vi "06_2.vi"() -> ()   [LabVIEW 2018]
uses:
  <userlib>/_OpenG.lib/array/array.llb/Search 1D Array (U8)__ogtk.vi
panel:
  out "sum":i16
  in  "String":string="wzaopvscxknyjtiul\nbelforsgdhuvmwc\n\nkiocpzjhsetqnwbl\nmaciywlbpodgevujnsktrz\nkpebjfchtlsonwiz\npcezwjtsinxlobk\n\nlrcp\ncdlbepr\nrlqcyutp\nlcpr\nlrtcpym\n\ngxcqbowaelfjhpknz\ngflhackzwqxojeb\nlfwocexqbkjhgaz\n\nfpivaozqnkextmbrjhycdwug\nmotgcrzaisqlpdwbeyhukf\nhbiqcdmkpawueyztgfor\nzrcehkqyoblmtgfiaupdw\n\numjz\njzu\nvzowkpuj\njmzau\n\nunzlx\nlnzxu\nmxluzn\nnzuxli\n\nszkiauhyntdrbcljomqwepv\namowcpzbyukihsjtqelnd\nlzctuqjabmsynphkewxido\nsikblhptcoqemdanywzju\njdeiylutspabcwngfzqkhom\n\nzgyhwtnxjdqucbp\nptnzhudjbcxgkqf\nzgqhjbdnutcmpx\ngjbzhpdxanqcut\n\nwjkcsqlu\nucsjq\n\nvkzsqtunmr\nljcexadhg\n\nfhtrusba\nsvtk\npgzwytn\nastb\n\nhvzjiwlsmnatbxg..."
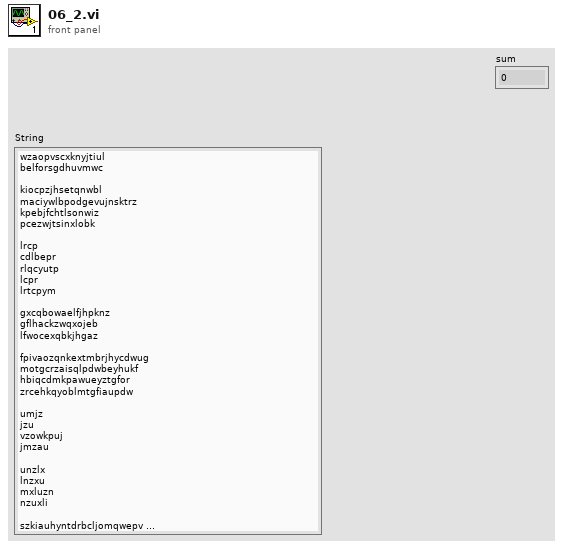
[diagram p1: front panel]
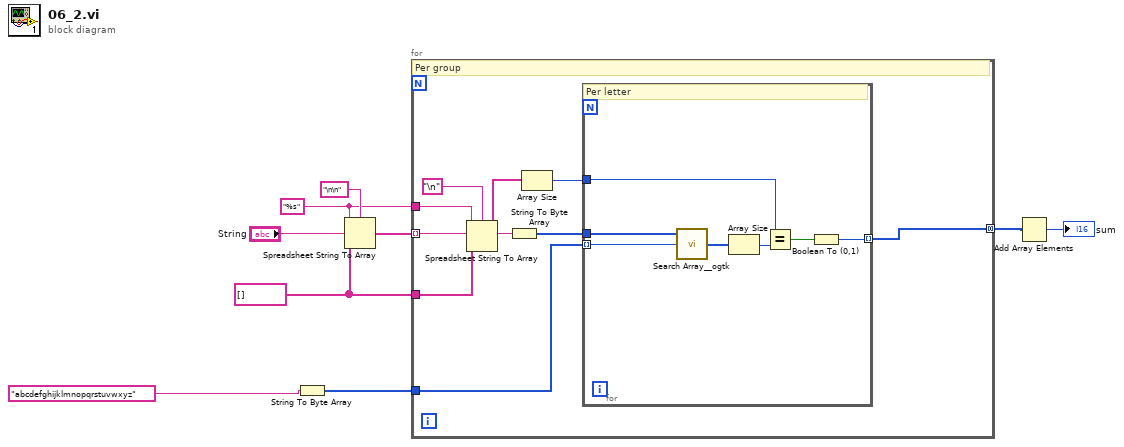
[diagram p0: block diagram]
diagram:
  w3 = string[] []
  w4 = "%s"
  n1 = String To Byte Array(string="abcdefghijklmnopqrstuvwxyz") -> (unsigned byte array=w1:u8[])
  n2 = Spreadsheet String To Array(delimiter (Tab)="\n\n", format string=w4, spreadsheet string="String", array type (2D Dbl)=w3) -> (array=w7:string[])
  n3 = for {
    tunnel: w7 -> [w14] mode=indexing
    tunnel: [w11] -> w6 mode=concatenating
    tunnel: w4 -> [w18]
    tunnel: w3 -> [w16]
    tunnel: w1 -> [w10]
    # "Per group"
    n4 = Spreadsheet String To Array(delimiter (Tab)="\n", format string=w18, spreadsheet string=w14, array type (2D Dbl)=w16) -> (array=w15:string[])
    n5 = String To Byte Array(string=w14) -> (unsigned byte array=w13:u8[])
    n6 = Array Size(array=w15) -> (size(s)=w12:i32)
    n7 = for {
      tunnel: w13 -> [w25]
      tunnel: w12 -> [w22]
      tunnel: [w20] -> w11 mode=indexing
      tunnel: w10 -> [w19] mode=indexing
      # "Per letter"
      n8 = call-poly <userlib>:"Search Array__ogtk.vi"("Array"=w25, "Element Data"=w19) -> ("Indices of Elements"=w24:i32[])  [unwired: 7 in]
      n9 = Array Size(array=w24) -> (size(s)=w23:i32)
      n10 = Equal?(x=w22, y=w23) -> (x = y?=w21:bool)
      n11 = Boolean To (0,1)(Boolean=w21) -> (0, 1=w20:i16)
    }
  }
  n12 = Add Array Elements(numeric array=w6) -> (sum=→"sum":i16)
